vi "Data2Graph.vi"(2 "length":i32, 3 "queue in":refnum<queue>, 4 "时域？":bool, 5 "element":dbl) -> (0 "subarray":dbl[](array[numeric]), 1 "queue out":refnum<queue>)   [LabVIEW 2014]
uses:
  <vilib>/Analysis/2dsp.llb/Real FFT.vi
  <vilib>/Analysis/NI_AALPro.lvlib
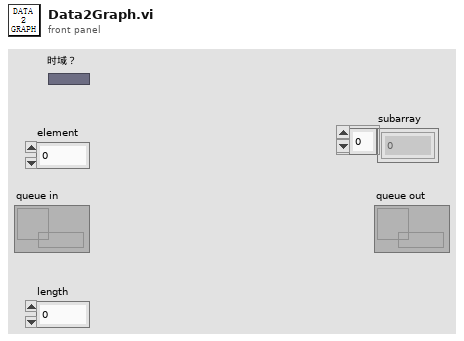
[diagram p1: front panel]
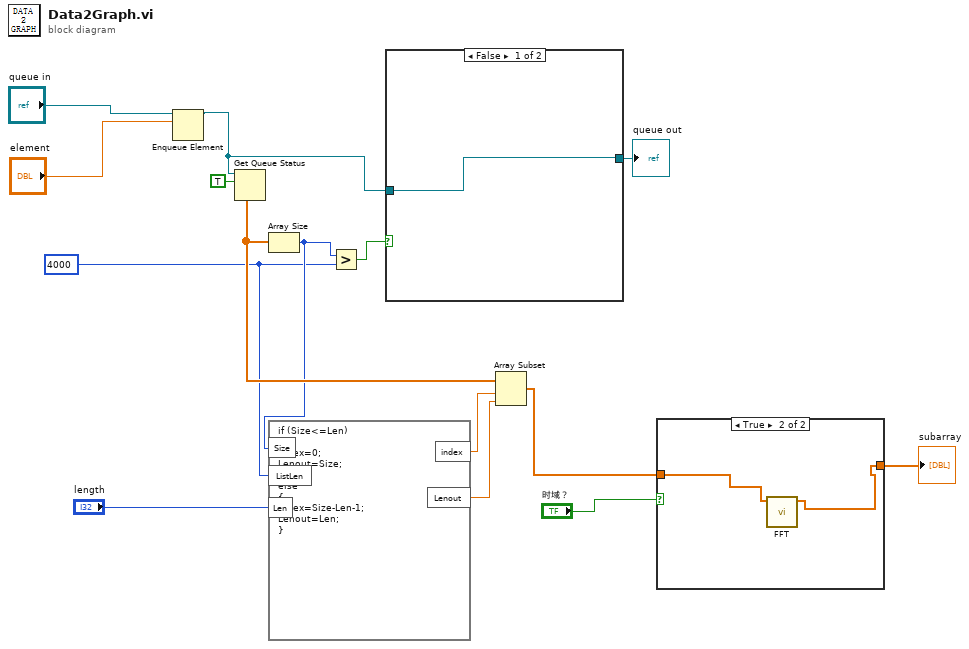
[diagram p0: block diagram]
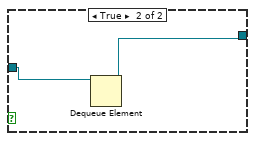
[diagram p3: hidden frame]
diagram:
  w7 = 4000
  n1 = Enqueue Element(queue="queue in", element="element") -> (queue out=w13:refnum<queue>)  [unwired: 2 in, 2 out]
  n2 = Get Queue Status(queue=w13, return elements? (F)=TRUE) -> (elements=w9:dbl[])  [unwired: 1 in, 7 out]
  n3 = Array Size(array=w9) -> (size(s)=w8:i32)
  n4 = formula code="if (Size<=Len)\n{\nindex=0;\nLenout=Size;\n}\nelse\n{\nindex=Size-Len-1;\nLenout=Len;\n}"("Size"=w8, "ListLen"=w7, "Len"="length") -> ("index"=w5:dbl, "Lenout"=w4:dbl)
  n5 = Greater?(x=w8, y=w7) -> (0:w14:bool)
  n6 = case shown="False" w14 {
    tunnel: w13 -> [w16 w18]
    tunnel: [w16 w17] -> w11
    frame False {
    }
    frame True {
      n7 = Dequeue Element(queue=w18) -> (queue out=w17:refnum<queue>)  [unwired: 2 in, 3 out]
    }
  }
  "queue out" <- w11
  n8 = Array Subset(array=w9, index=w5, length=w4) -> (w2:dbl[])
  n9 = case shown="True" "时域？" {
    tunnel: w2 -> [w19 w21]
    tunnel: [w19 w20] -> w1
    frame False {
    }
    frame True {
      n10 = call-poly <vilib>:"FFT.vi"("X"=w21) -> ("FFT {X}"=w20:cdb[])  [unwired: 9 in, 1 out]
    }
  }
  "subarray" <- w1
